vi "Agilent PWM Set Offset Value.vi"(7 "Agilent PWM":T1, 8 "error in (no error)":errorcluster, 10 "Offset Value (dBm)":dbl, 11 "VISA Resource Name":refnum<visa-resource-name>) -> (0 "error out":errorcluster, 3 "dup VISA Resource Name":refnum<visa-resource-name>)   [LabVIEW 2011]
doc: "This VI for the HP 8753 is used to read the sweep type.\n\n0 LINEAR FREQ\n1 LOG FREQ\n2 LIST FREQ\n3 CW TIME\n4 POWER SWEEP"
uses:
  TypeDefs/Agilent PWM Instrument Info.ctl
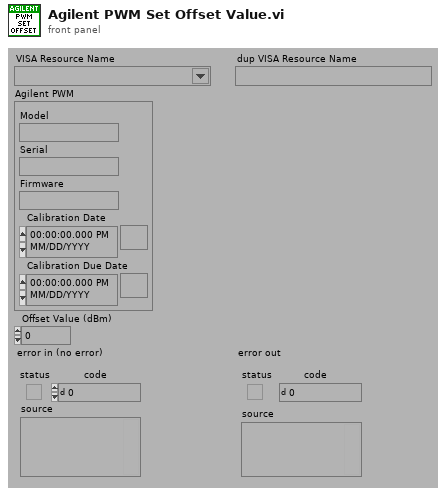
[diagram p1: front panel]
types:
  T1 = typedef "Agilent PWM Instrument Info.ctl" = cluster{"Model":string, "Serial":string, "Firmware":string, "Calibration Date":timestamp, "Calibration Due Date":timestamp}
  T2 = typedef "Agilent PWM Model.ctl" = enum16{"Not Supported", "E4418X", "E4419X", "U2000X"}
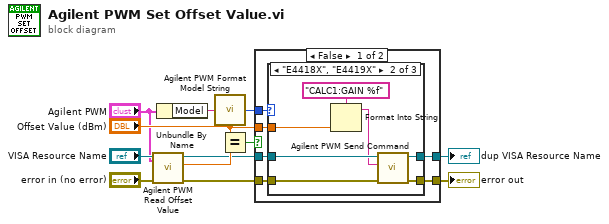
[diagram p0: block diagram]
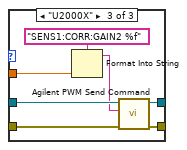
[diagram p3: hidden frame]
diagram:
  n1 = call "Agilent PWM Read Offset Value.vi"("Agilent PWM"="Agilent PWM", "error in (no error)"="error in (no error)", "VISA Resource Name"="VISA Resource Name") -> ("error out"=w8:errorcluster, "Value (dB)"=w10:dbl, "dup VISA Resource Name"=w7:refnum<visa-resource-name>)  [unwired: 6 out]
  n2 = Unbundle By Name("Agilent PWM") -> ("Model"=w9:string)
  n3 = call "Agilent PWM Format Model String.vi"("Model"=w9) -> ("Model"=w3:T2)
  n4 = Equal?(x="Offset Value (dBm)", y=w10) -> (x = y?=w1:bool)
  n5 = case shown="False" w1 {
    tunnel: [w18 w36] -> w6
    tunnel: [w17 w35] -> w5
    tunnel: w7 -> [w16 w36]
    tunnel: w8 -> [w15 w35]
    tunnel: "Offset Value (dBm)" -> [w14 _]
    tunnel: w3 -> [w13 _]
    frame False {
      n6 = case shown="\"E4418X\", \"E4419X\"" w13 {
        tunnel: [w20 w27 w34] -> w18
        tunnel: [w19 w26 w33] -> w17
        tunnel: w16 -> [w20 w25 w32]
        tunnel: w15 -> [w19 w24 w31]
        tunnel: w14 -> [_ w21 w28]
        frame "Not Supported" {
        }
        frame "E4418X", "E4419X" {
          n7 = Format Into String(format string="CALC1:GAIN %f" ("write buffer"), w21) -> (resulting string=w22:string)  [unwired: 2 in, 1 out]
          n8 = call "Agilent PWM Send Command.vi"("error in (no error)"=w24, "Command"=w22, "VISA Resource Name"=w25) -> ("error out"=w26:errorcluster, "dup VISA Resource Name"=w27:refnum<visa-resource-name>)  [unwired: 2 in, 5 out]
        }
        frame "U2000X" {
          n9 = Format Into String(format string="SENS1:CORR:GAIN2 %f" ("write buffer"), w28) -> (resulting string=w29:string)  [unwired: 2 in, 1 out]
          n10 = call "Agilent PWM Send Command.vi"("error in (no error)"=w31, "Command"=w29, "VISA Resource Name"=w32) -> ("error out"=w33:errorcluster, "dup VISA Resource Name"=w34:refnum<visa-resource-name>)  [unwired: 2 in, 5 out]
        }
      }
    }
    frame True {
    }
  }
  "dup VISA Resource Name" <- w6
  "error out" <- w5
